vi "MMEM_DAT-FLAG.vi"(0 "PNA IN":refnum<visa-resource-name>="TCPIP0::169.254.70.180::inst0::INSTR", 1 "FilePath":string="D:\\State Files\\WAM_PRODUCTION.csa", 5 "error in":errorcluster, 7 "PopUp Alert(t)":bool, 9 "HrsToFlag":dbl=24.0) -> (6 "CalMessage":string, 8 "=>SelectedHrs?(t)":bool=TRUE, 10 "system time(str)":string, 12 "File Time/Date Out (Str)":string, 14 "VISA Out":refnum<visa-resource-name>="TCPIP0::169.254.70.180::inst0::INSTR", 19 "error out":errorcluster)   [LabVIEW 2018]
doc: "Reads the selected file last modified daye/time.\n\nThen will compare to a preset flag in HRs."
panel:
  out "Hrs":string
  out "file time":timestamp
  out "HRS DIFF":dbl=0.9993685132927365
  out "pna time":timestamp=timestamp(3761139683 s since 1904-01-01) format="%<%X\n%x>T"
  out "PNA-DATE/TIME":string="13:01:23 03/08/2023 "
  out "system time":timestamp=timestamp(3761143280.726648 s since 1904-01-01) format="%<%X\n%x>T"
  # "This vi will check the age of a file and throw a flag if the file is older than HRS specified"
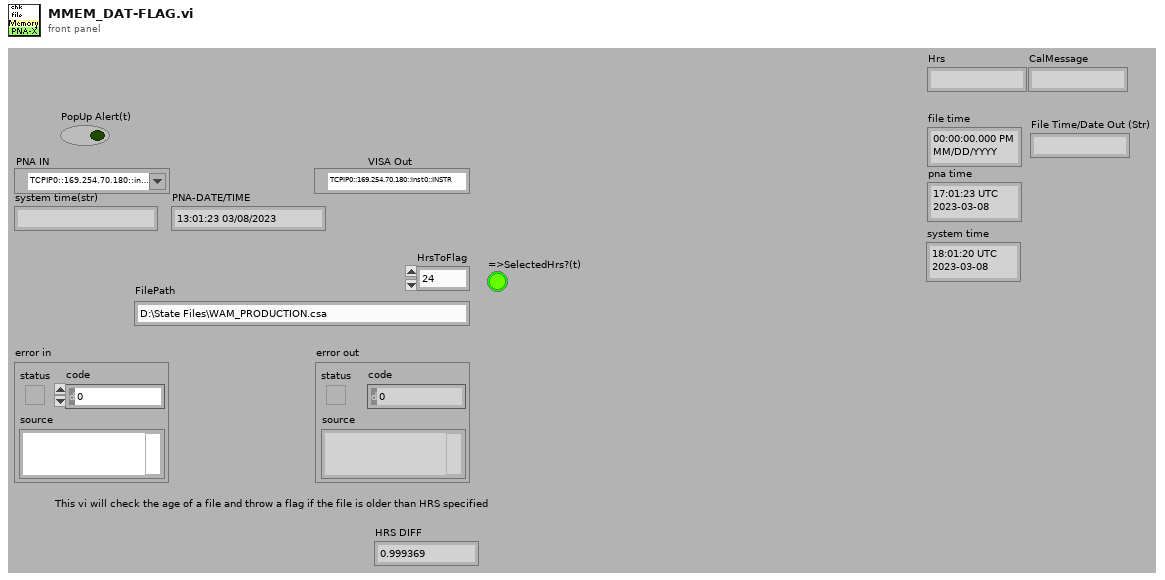
[diagram p1: front panel]
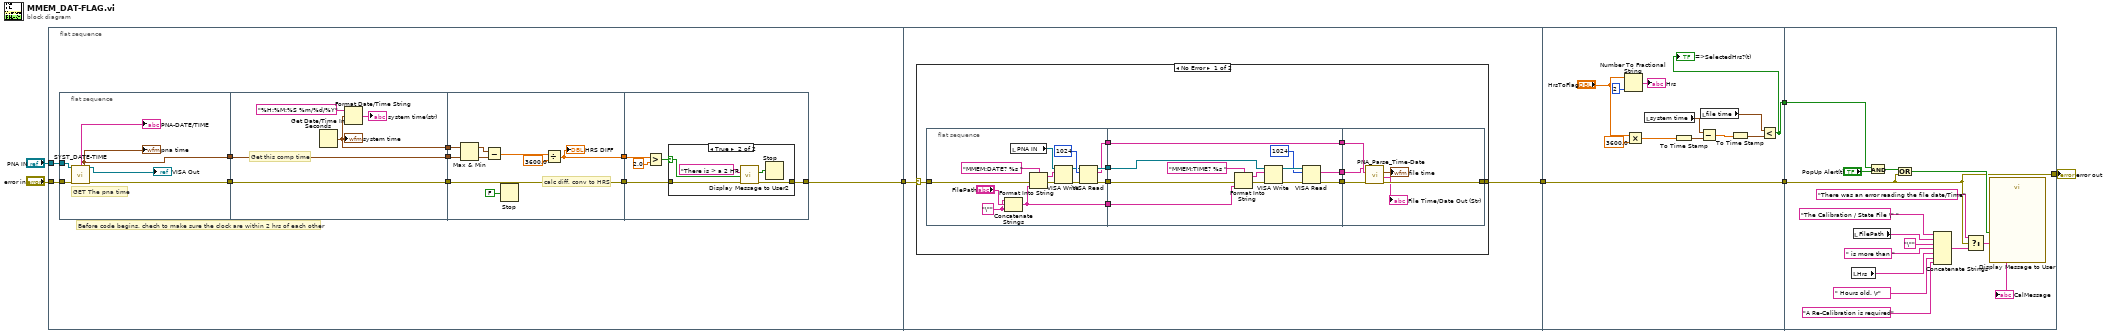
[diagram p0: block diagram]
diagram:
  n1 = flat-sequence {
    tunnel: "PNA IN" -> [w17]
    tunnel: "error in" -> [w16]
    tunnel: [w15] -> w4
    tunnel: [w49] -> w3
    tunnel: w4 -> [w50]
    tunnel: w3 -> [w104]
    tunnel: [w104] -> w2
    tunnel: [w96] -> w1
    tunnel: [w106] -> w6
    tunnel: w2 -> [w106]
    tunnel: w1 -> [w119]
    frame #0 {
      # "Before code begins, chech to make sure the clock are within 2 hrs of each other"
      n2 = flat-sequence {
        tunnel: w17 -> [w23]
        tunnel: w16 -> [w22]
        tunnel: [w21] -> w14
        tunnel: [w19] -> w11
        tunnel: w14 -> [w28]
        tunnel: [w28] -> w13
        tunnel: [w26] -> w12
        tunnel: w11 -> [w27]
        tunnel: [w27] -> w10
        tunnel: w13 -> [w37]
        tunnel: w12 -> [w32]
        tunnel: w10 -> [w31]
        tunnel: [w37] -> w9
        tunnel: [w30] -> w8
        tunnel: [w39] -> w15
        tunnel: w9 -> [w40]
        tunnel: w8 -> [w42]
        frame #0 {
          # "GET The pna time"
          n3 = call "SYST_DATE-TIME.vi"("Session In"=w23, "error in"=w22) -> ("Date/Time(str)"=→"PNA-DATE/TIME":string, "timestamp"=w19:timestamp, "Session Out"=→"VISA Out":refnum<visa-resource-name>, "error out"=w21:errorcluster)  [unwired: 10 in]
          "pna time" <- w19
        }
        frame #1 {
          # "Get this comp time"
          n4 = Get Date/Time In Seconds() -> (seconds since 1Jan1904=w26:timestamp)
          "system time" <- w26
          n5 = Format Date/Time String(time format string (%c)="%H:%M:%S %m/%d/%Y", seconds (now)=w26) -> (date/time string=→"system time(str)":string)  [unwired: 1 in]
        }
        frame #2 {
          # "calc diff, conv to HRS"
          n6 = Max & Min(x=w32, y=w31) -> (max(x,y)=w34:timestamp, min(x,y)=w35:timestamp)
          n7 = Subtract(x=w34, y=w35) -> (x-y=w36:dbl)
          n8 = Stop(stop? (T)=FALSE) -> ()
          n9 = Divide(x=w36, y=3600.0) -> (x/y=w30:dbl)
          "HRS DIFF" <- w30
        }
        frame #3 {
          n10 = Greater?(x=w42, y=2.0) -> (0:w38:bool)
          n11 = case shown="True" w38 {
            selector: w38 -> [_ w44]
            tunnel: w40 -> [w43 w48]
            tunnel: [w43 w47] -> w39
            frame False {
            }
            frame True {
              n12 = call "Display Message to User2"("error in (no error)"=w48, "Enable"=w44, "Message"="There is > a 2 HR time difference between the PNA clock and the Computer system clock") -> ("error out"=w47:errorcluster, "OK[Continue]"=w45:bool)  [unwired: 7 in]
              n13 = Stop(stop? (T)=w45) -> ()
            }
          }
        }
      }
    }
    frame #1 {
      n14 = case shown="No Error" w50 {
        selector: w50 -> [w59 w92]
        tunnel: [w52 w92] -> w49
        frame No Error {
          n15 = flat-sequence {
            tunnel: w59 -> [w73]
            tunnel: [w64] -> w58
            tunnel: [w63] -> w57
            tunnel: [w62] -> w56
            tunnel: [w61] -> w55
            tunnel: w58 -> [w76]
            tunnel: w57 -> [w79]
            tunnel: w56 -> [w77]
            tunnel: w55 -> [w85]
            tunnel: [w85] -> w54
            tunnel: [w75] -> w53
            tunnel: [w74] -> w51
            tunnel: w54 -> [w90]
            tunnel: w53 -> [w89]
            tunnel: [w88] -> w52
            tunnel: w51 -> [w87]
            frame #0 {
              w65 = "\"" ("string")
              n16 = Concatenate Strings(w65, "FilePath", w65) -> (w64:string)
              n17 = local read "PNA IN"() -> (w60:refnum<visa-resource-name>)
              n18 = Format Into String(format string="MMEM:DATE? %s " ("Cmdline"), error in=w73, w64) -> (resulting string=w71:string, error out=w72:errorcluster)  [unwired: 1 in]
              n19 = VISA Write(VISA resource name=w60, write buffer=w71, error in (no error)=w72) -> (VISA resource name out=w67:refnum<visa-resource-name>, error out=w69:errorcluster)  [unwired: 1 out]
              n20 = VISA Read(VISA resource name=w67, byte count=1024, error in (no error)=w69) -> (VISA resource name out=w63:refnum<visa-resource-name>, read buffer=w61:string, error out=w62:errorcluster)  [unwired: 1 out]
            }
            frame #1 {
              n21 = Format Into String(format string="MMEM:TIME? %s " ("Cmdline"), error in=w77, w76) -> (resulting string=w83:string, error out=w84:errorcluster)  [unwired: 1 in]
              n22 = VISA Write(VISA resource name=w79, write buffer=w83, error in (no error)=w84) -> (VISA resource name out=w81:refnum<visa-resource-name>, error out=w82:errorcluster)  [unwired: 1 out]
              n23 = VISA Read(VISA resource name=w81, byte count=1024, error in (no error)=w82) -> (read buffer=w75:string, error out=w74:errorcluster)  [unwired: 2 out]
            }
            frame #2 {
              n24 = call "PNA_Parse_Time-Date.vi"("error in (no error)"=w87, "SYST:DATE (IN)"=w90, "SYST:TIME (IN)"=w89) -> ("error out"=w88:errorcluster, "Time/Date Out (Str)"=→"File Time/Date Out (Str)":string, "Time Stamp"=→"file time":timestamp)  [unwired: 4 in, 2 out]
            }
          }
        }
        frame Error {
        }
      }
    }
    frame #2 {
      n25 = Number To Fractional String(number="HrsToFlag", precision (6)=i16 2) -> (F-format string=→"Hrs":string)  [unwired: 2 in]
      n26 = Multiply(x="HrsToFlag", y=3600.0) -> (x*y=w101:dbl)
      n27 = local read "system time"() -> (w102:timestamp)
      n28 = To Time Stamp(1:w101) -> (0:w99:timestamp)
      n29 = Subtract(x=w102, y=w99) -> (x-y=w100:dbl)
      n30 = local read "file time"() -> (w103:timestamp)
      n31 = To Time Stamp(1:w100) -> (0:w98:timestamp)
      n32 = Less?(x=w103, y=w98) -> (x < y?=w96:bool)
      "=>SelectedHrs?(t)" <- w96
    }
    frame #3 {
      n33 = local read "Hrs"() -> (w105:string)
      n34 = local read "FilePath"() -> (w117:string)
      n35 = And(x=w119, y="PopUp Alert(t)") -> (x .and. y?=w112:bool)
      n36 = Or(x=w112, y=w106) -> (x .or. y?=w107:bool)
      n37 = Concatenate Strings("The Calibration / State File \" " ("string"), w117, "\"", " is more than ", w105, " Hours old. \r" ("string"), "A Re-Calibration is required" ("string")) -> (w108:string)
      n38 = Select(t="There was an error reading the file date/Time" ("f"), s=w106, f=w108) -> (s? t:f=w110:string)
      "CalMessage" <- w110
      n39 = call "Display Message to User"("Enable"=w107, "Message"=w110) -> ()  [unwired: 8 in, 2 out]
    }
  }
  "error out" <- w6
